vi "xml single result.vi"(6 "limit type":enum16{"上限", "下限"}(ring), 7 "ABS?":bool, 8 "second result":string, 9 "single spec":dbl[](array[numeric]), 10 "TX data":string[](array[string]), 11 "RX data":string[](array[string])) -> (2 "TX array":string[](array[string]), 3 "RX array":string[](array[string]))   [LabVIEW 2011]
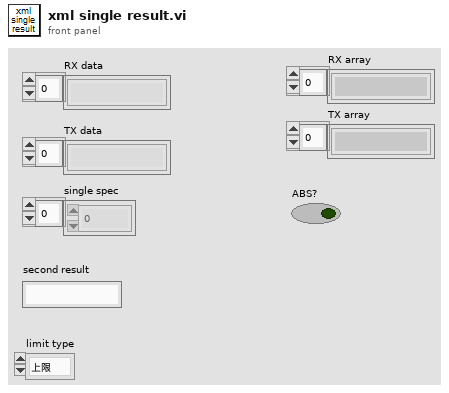
[diagram p1: front panel]
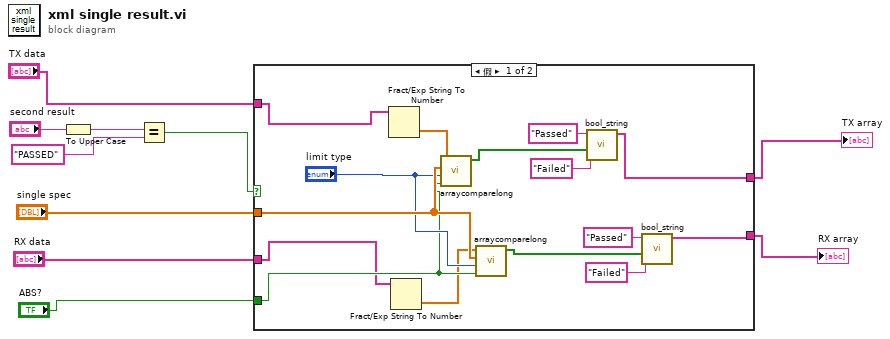
[diagram p0: block diagram]
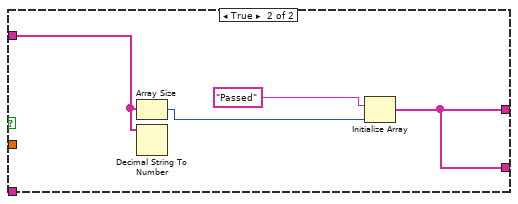
[diagram p2: hidden frame]
diagram:
  n1 = To Upper Case(1:"second result") -> (0:w9:string)
  n2 = Equal?(x=w9, y="PASSED") -> (x = y?=w7:bool)
  n3 = case shown="假" w7 {
    tunnel: "TX data" -> [w14 w27]
    tunnel: [w23 w26] -> w2
    tunnel: [w20 w26] -> w1
    tunnel: "RX data" -> [w12 _]
    tunnel: "single spec" -> [w18 _]
    tunnel: "ABS?" -> [w15 _]
    frame False {
      n4 = Fract/Exp String To Number(string=w14) -> (number=w13:dbl[])  [unwired: 3 in, 1 out]
      n5 = Fract/Exp String To Number(string=w12) -> (number=w11:dbl[])  [unwired: 3 in, 1 out]
      n6 = call "arraycomparelong.vi"("ABS?"=w15, "limit type"="limit type", "spec"=w18, "data"=w13) -> ("result"=w19:bool[])  [unwired: 7 in]
      n7 = call "arraycomparelong.vi"("ABS?"=w15, "limit type"="limit type", "spec"=w18, "data"=w11) -> ("result"=w17:bool[])  [unwired: 7 in]
      n8 = call "bool_string.vi"("boolean array"=w19, "FalseValue"="Failed", "TrueValue"="Passed") -> ("string array"=w23:string[])  [unwired: 8 in]
      n9 = call "bool_string.vi"("boolean array"=w17, "FalseValue"="Failed", "TrueValue"="Passed") -> ("string array"=w20:string[])  [unwired: 8 in]
    }
    frame True {
      n10 = Array Size(array=w27) -> (size(s)=w28:i32)
      n11 = Decimal String To Number(string=w27) -> ()  [unwired: 2 in, 2 out]
      n12 = Initialize Array("Passed" ("y"), w28) -> (w26:string[])
    }
  }
  "RX array" <- w1
  "TX array" <- w2
